vi "Example Creation of JSON string.vi"() -> ()   [LabVIEW 2011]
doc: "Building up of a complex JSON from smaller units"
uses:
  vi.lib/Addons/JSON API/JSON Object/JSON Object.lvclass
  vi.lib/Addons/JSON API/JSON Object/Set Object Item by name.vi
  vi.lib/Addons/JSON API/JSON Array/Set JSON Array.vi
  vi.lib/Addons/JSON API/JSON Scalar/Set DBL.vi
  vi.lib/Addons/JSON API/JSON Scalar/Set String.vi
  vi.lib/Addons/JSON API/JSON Scalar/Set Timestamp.vi
  vi.lib/Addons/JSON API/JSON Value/Get as JSON string (pretty).vi
  vi.lib/Addons/JSON API/JSON Scalar/JSON Scalar.lvclass
  vi.lib/Addons/JSON API/Get Polymorphic/JSON GetSet.lvlib
  vi.lib/Addons/JSON API/JSON Array/JSON Array.lvclass
  vi.lib/Addons/JSON API/JSON Value/JSON Value.lvclass
panel:
  out "JSON":string
  # "see diagram"
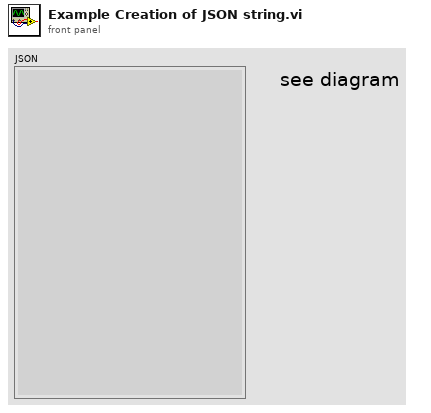
[diagram p1: front panel]
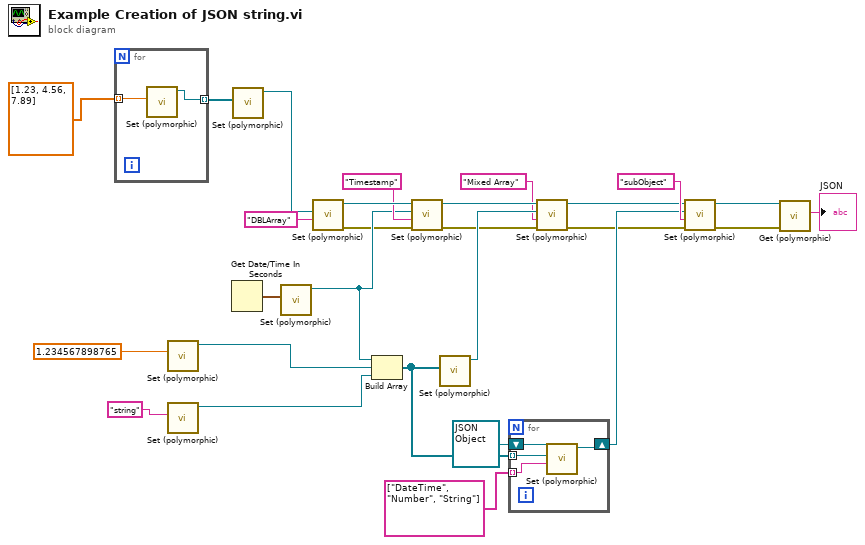
[diagram p0: block diagram]
diagram:
  n1 = for {
    tunnel: dbl[] [1.23, 4.56, 7.89] -> [w29] mode=indexing
    tunnel: [w28] -> w26 mode=indexing
    n2 = call-poly "Set (polymorphic).vi"("Numeric"=w29) -> ("JSON Scalar out"=w28:refnum<class "JSON Scalar.lvclass">)  [unwired: 9 in, 1 out]
  }
  n3 = call-poly "Set (polymorphic).vi"("Numeric"=1.234567898765) -> ("JSON Scalar out"=w17:refnum<class "JSON Scalar.lvclass">)  [unwired: 9 in, 1 out]
  n4 = call-poly "Set (polymorphic).vi"("String"="string") -> ("JSON Scalar out"=w16:refnum<class "JSON Scalar.lvclass">)  [unwired: 9 in, 1 out]
  n5 = Get Date/Time In Seconds() -> (seconds since 1Jan1904=w22:timestamp)
  n6 = call-poly "Set (polymorphic).vi"("Array"=w26) -> ("JSON Array out"=w25:refnum<class "JSON Array.lvclass">)  [unwired: 9 in, 1 out]
  n7 = call-poly "Set (polymorphic).vi"("Time Stamp"=w22) -> ("JSON Scalar out"=w18:refnum<class "JSON Scalar.lvclass">)  [unwired: 9 in, 1 out]
  n8 = call-poly "Set (polymorphic).vi"("name"="DBLArray", "Value"=w25) -> ("error out"=w11:errorcluster, "JSON Object out"=w23:refnum<class "JSON Object.lvclass">)  [unwired: 7 in, 1 out]
  n9 = Build Array(w18, w17, w16) -> (w10:refnum<class "JSON Scalar.lvclass">[])
  n10 = call-poly "Set (polymorphic).vi"("error in (no error)"=w11, "name"="Timestamp", "Value"=w18, "JSON Object in"=w23) -> ("error out"=w12:errorcluster, "JSON Object out"=w15:refnum<class "JSON Object.lvclass">)  [unwired: 5 in, 1 out]
  n11 = call-poly "Set (polymorphic).vi"("Array"=w10) -> ("JSON Array out"=w14:refnum<class "JSON Array.lvclass">)  [unwired: 9 in, 1 out]
  n12 = for {
    tunnel: w10 -> [w33] mode=indexing
    shift-right: [w31] -> w5
    shift-left: refnum<class "JSON Object.lvclass"> refnum ("JSON Object out") -> [w32]
    tunnel: string[] ["DateTime", "Number", "String"] -> [w30] mode=indexing
    n13 = call-poly "Set (polymorphic).vi"("name"=w30, "Value"=w33, "JSON Object in"=w32) -> ("JSON Object out"=w31:refnum<class "JSON Object.lvclass">)  [unwired: 6 in, 2 out]
  }
  n14 = call-poly "Set (polymorphic).vi"("error in (no error)"=w12, "name"="Mixed Array", "Value"=w14, "JSON Object in"=w15) -> ("error out"=w2:errorcluster, "JSON Object out"=w6:refnum<class "JSON Object.lvclass">)  [unwired: 5 in, 1 out]
  n15 = call-poly "Set (polymorphic).vi"("error in (no error)"=w2, "name"="subObject", "Value"=w5, "JSON Object in"=w6) -> ("error out"=w3:errorcluster, "JSON Object out"=w4:refnum<class "JSON Object.lvclass">)  [unwired: 5 in, 1 out]
  n16 = call-poly "Get (polymorphic).vi"("error in (no error)"=w3, "JSON Value in"=w4) -> ("String"=→"JSON":string)  [unwired: 8 in, 1 out]
